vi "get index definition.vi"(10 "channel classification":T1, 11 "GPIC ScaleAndLimit configuration in":refnum<class "GPIC ScaleAndLimit configuration.lvclass">) -> (1 "valid?":bool, 2 "index cluster":variant, 3 "GPIC ScaleAndLimit configuration out":refnum<class "GPIC ScaleAndLimit configuration.lvclass">)   [LabVIEW 2015, in "GPIC ScaleAndLimit configuration.lvclass"]
uses:
  GPIC ScaleAndLimit configuration.lvclass
  <vilib>/NI/Tag Bus Module Framework/channel/channel classification.ctl
  input data indices.ctl
  output data indices.ctl
  parameter data indices.ctl
  result data indices.ctl
  <vilib>/NI/Tag Bus Module Framework/channel/TBM channel.lvclass
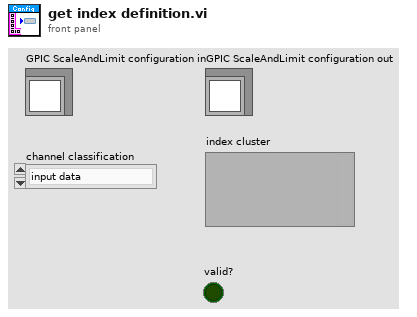
[diagram p1: front panel]
types:
  T1 = typedef "TBM channel.lvclass/channel classification.ctl" = enum16{"input data", "output data", "processing parameter", "processing result"}
  T2 = typedef "GPIC ScaleAndLimit configuration.lvclass/input data indices.ctl" = cluster{"Single.RMC/Simultaneous/AI0":i32, "Single.RMC/Simultaneous/AI1":i32, "Single.RMC/Simultaneous/AI2":i32, "Single.RMC/Simultaneous/AI3":i32, "Single.RMC/Simultaneous/AI4":i32, "Single.RMC/Simultaneous/AI5":i32, "Single.RMC/Simultaneous/AI6":i32, "Single.RMC/Simultaneous/AI7":i32, "Single.RMC/Simultaneous/AI8":i32, "Single.RMC/Simultaneous/AI9":i32, "Single.RMC/Simultaneous/AI10":i32, "Single.RMC/Simultaneous/AI11":i32, "Single.RMC/Simultaneous/AI12":i32, "Single.RMC/Simultaneous/AI13":i32, "Single.RMC/Simultaneous/AI14":i32, "Single.RMC/Simultaneous/AI15":i32, "Boolean.AILimits":i32, "U16.AILimitHigh":i32, "U16.AILimitLow":i32}
  T3 = typedef "GPIC ScaleAndLimit configuration.lvclass/output data indices.ctl" = cluster{"Boolean.ClearLimits":i32}
  T4 = typedef "GPIC ScaleAndLimit configuration.lvclass/parameter data indices.ctl" = cluster{"fmwk_placeholder":i32}
  T5 = typedef "GPIC ScaleAndLimit configuration.lvclass/result data indices.ctl" = cluster{"fmwk_placeholder":i32}
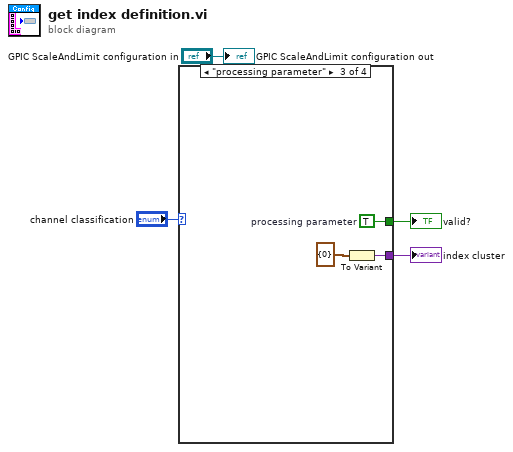
[diagram p0: block diagram]
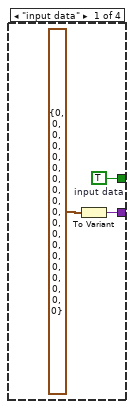
[diagram p2: hidden frame]
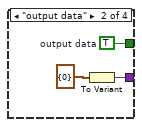
[diagram p3: hidden frame]
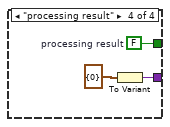
[diagram p4: hidden frame]
diagram:
  n1 = case shown="\"processing parameter\"" "channel classification" {
    tunnel: [w6 w10 w13 w16] -> w2
    tunnel: [w5 w9 w12 w15] -> w1
    frame "input data" {
      w5 = TRUE  # input data
      n2 = To Variant(anything=T2 {"Single.RMC/Simultaneous/AI0"=0, "Single.RMC/Simultaneous/AI1"=0, "Single.RMC/Simultaneous/AI2"=0, "Single.RMC/Simultaneous/AI3"=0, "Single.RMC/Simultaneous/AI4"=0, "Single.RMC/Simultaneous/AI5"=0, "Single.RMC/Simultaneous/AI6"=0, "Single.RMC/Simultaneous/AI7"=0, "Single.RMC/Simultaneous/AI8"=0, "Single.RMC/Simultaneous/AI9"=0, "Single.RMC/Simultaneous/AI10"=0, "Single.RMC/Simultaneous/AI11"=0, "Single.RMC/Simultaneous/AI12"=0, "Single.RMC/Simultaneous/AI13"=0, "Single.RMC/Simultaneous/AI14"=0, "Single.RMC/Simultaneous/AI15"=0, "Boolean.AILimits"=0, "U16.AILimitHigh"=0, "U16.AILimitLow"=0} ("Cluster")) -> (Variant=w6:variant)
    }
    frame "output data" {
      w9 = TRUE  # output data
      n3 = To Variant(anything=T3 {"Boolean.ClearLimits"=0} ("Cluster")) -> (Variant=w10:variant)
    }
    frame "processing parameter" {
      w12 = TRUE  # processing parameter
      n4 = To Variant(anything=T4 {"fmwk_placeholder"=0} ("Cluster")) -> (Variant=w13:variant)
    }
    frame "processing result" {
      w15 = FALSE  # processing result
      n5 = To Variant(anything=T5 {"fmwk_placeholder"=0} ("Cluster")) -> (Variant=w16:variant)
    }
  }
  "index cluster" <- w2
  "valid?" <- w1
  "GPIC ScaleAndLimit configuration out" <- "GPIC ScaleAndLimit configuration in"
